vi "DIO In Get (Water Tank).vi"(8 "error in (no error)":errorcluster, 11 "DigitalInputDevRef":cluster{string, i32}) -> (0 "error out":errorcluster, 2 "Value":bool, 3 "DigitalInputDevRef":cluster{string, i32})   [LabVIEW 2013]
uses:
  Water Tank Global.vi
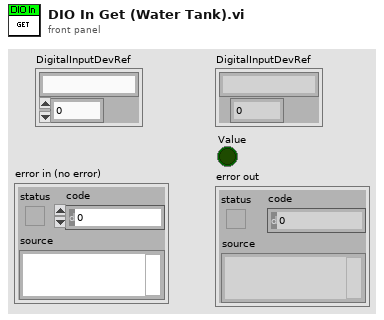
[diagram p1: front panel]
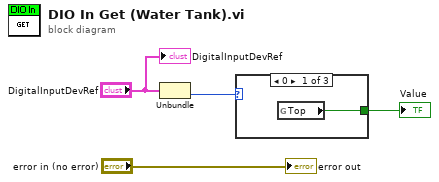
[diagram p0: block diagram]
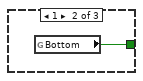
[diagram p2: hidden frame]
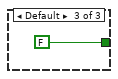
[diagram p3: hidden frame]
diagram:
  n1 = Unbundle("DigitalInputDevRef") -> (w2:i32)  [unwired: 1 out]
  n2 = case shown="0" w2 {
    tunnel: [w5 w6 FALSE] -> w1
    frame 0 {
      n3 = global read "Water Tank Global.vi" "Top"() -> (w5:bool)
    }
    frame 1 {
      n4 = global read "Water Tank Global.vi" "Bottom"() -> (w6:bool)
    }
    frame Default {
    }
  }
  "Value" <- w1
  "error out" <- "error in (no error)"
  "DigitalInputDevRef" <- "DigitalInputDevRef"
